vi "getYearMonthString.vi"(8 "error in (no error)":errorcluster, 11 "WhichMonth in":refnum<class "WhichMonth.lvclass">) -> (0 "error out":errorcluster, 2 "Year-Month":string, 3 "WhichMonth out":refnum<class "WhichMonth.lvclass">)   [LabVIEW 2018, in "WhichMonth.lvclass"]
uses:
  WhichMonth.lvclass
  WhichMonth.lvclass/WhichMonth.ctl
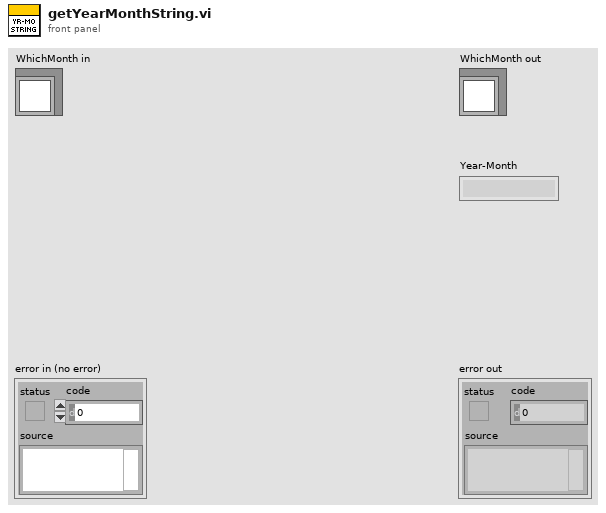
[diagram p1: front panel]
types:
  T1 = typedef "WhichMonth.lvclass/Month.ctl" = enum16{"January", "February", "March", "April", "May", "June", "July", "August", "September", "October", "November", "December"}
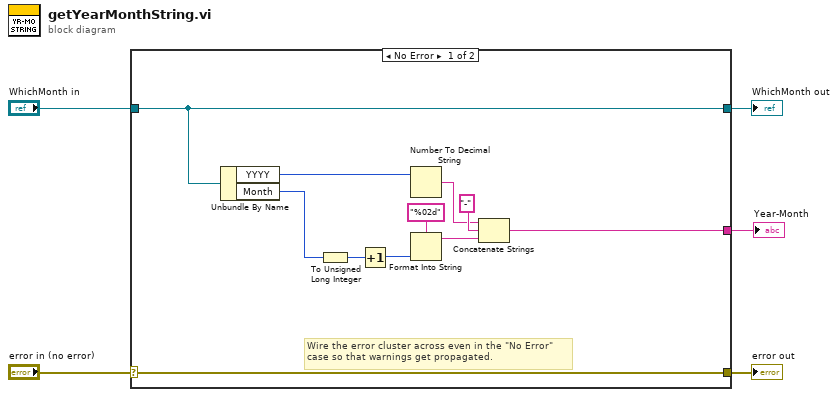
[diagram p0: block diagram]
diagram:
  n1 = case shown="No Error" "error in (no error)" {
    selector: "error in (no error)" -> [w16 w18]
    tunnel: [w16 w18] -> w4
    tunnel: [w9 w17] -> w2
    tunnel: "WhichMonth in" -> [w9 w17]
    tunnel: [w6 _] -> w1
    frame No Error {
      # "Wire the error cluster across even in the \"No Error\"\ncase so that warnings get propagated."
      n2 = Unbundle By Name(w9) -> ("YYYY"=w8:i32, "Month"=w7:T1)
      n3 = To Unsigned Long Integer(number=w7) -> (unsigned 32bit integer=w11:u32)
      n4 = Increment(x=w11) -> (x+1=w10:u32)
      n5 = Number To Decimal String(number=w8) -> (decimal integer string=w12:string)  [unwired: 1 in]
      n6 = Format Into String(format string="%02d" ("string"), w10) -> (resulting string=w14:string)  [unwired: 2 in, 1 out]
      n7 = Concatenate Strings(w12, "-" ("string"), w14) -> (w6:string)
    }
    frame Error {
    }
  }
  "error out" <- w4
  "WhichMonth out" <- w2
  "Year-Month" <- w1
